vi "Auto Info Globals.vi"() -> ()   [LabVIEW 2018]
panel:
  out "Platform 2?":bool
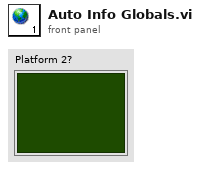
[diagram p1: front panel]
diagram:
